vi "Mouse Move.vi"(7 "Map Model in":refnum<class "Map Model.lvclass">, 8 "error in (no error)":errorcluster, 10 "Position":T1, 11 "Pencil in":refnum<class "Pencil.lvclass">) -> (0 "error out":errorcluster, 3 "Pencil out":refnum<class "Pencil.lvclass">, 5 "Map Model out":refnum<class "Map Model.lvclass">)   [LabVIEW 2020, in "Map Model.lvlib" / "Pencil.lvclass"]
uses:
  Pencil.lvclass
  E:/Project/Labview-Projects/Completed projects/Map Editor/Models/Map Model/Tools/Tool/Tool.lvclass
  <vilib>/Utility/miscctls.llb/LVPoint32TypeDef.ctl
  Map Model/Map Model.lvclass
  Tool/Tool.lvclass/Tool.ctl
  Map Model/Map Model.lvclass/Map Model.ctl
  Undoable Tool/Undoable Tool.lvclass
  Tool/Tool.lvclass
panel:
  # "NOTICE -- YOU MUST LEAVE THIS NOTICE IN PLACE.\n\nCopyright (c) 2017, LIANG LIU Shawn.Liu.cn@gmail.com\nAll rights reserved.\n\nRedistribution and use in source and binary forms, with or without modification, are permitted provided that the following conditions are met:\n-Redistributions of source code must retain the above copyright notice, this list of conditions and the following disclaimer.\n-Redistributions in binary form must reproduce the above copyright notice, this list of conditions and the following disclaimer in the documentation and/or other materials provided with the distribution.\n-Neither the name of the eLp nor the names of its contributors may be used to endorse or promote products derived from this software without specific prior written permission.\n\nTHIS SOFTWARE IS PROVIDED BY THE COPYRIGHT HOLDERS AND CONTRIBUTORS \"AS IS\" AND ANY EXPRESS OR IMPLIED WARRANTIES, INCLUDING, BUT NOT LIMITED TO, THE IMPLIED WARRANTIES OF MERCHANTABILITY AND FITNESS FOR A PARTICULAR PURPOSE ARE DISCLAIMED. IN NO EVENT SHALL THE COPYRIGHT HOLDER OR CONTRIBUTORS BE LIABLE FOR ANY DIRECT, INDIRECT, INCIDENTAL, SPECIAL, EXEMPLARY, OR CONSEQUENTIAL DAMAGES (INCLUDING, BUT NOT LIMITED TO, PROCUREMENT OF SUBSTITUTE GOODS OR SERVICES; LOSS OF USE, DATA, OR PROFITS; OR BUSINESS INTERRUPTION) HOWEVER CAUSED AND ON ANY THEORY OF LIABILITY, WHETHER IN CONTRACT, STRICT LIABILITY, OR TORT (INCLUDING NEGLIGENCE OR OTHERWISE) ARISING IN ANY WAY OUT OF THE USE OF THIS SOFTWARE, EVEN IF ADVISED OF THE POSSIBILITY OF SUCH DAMAGE."
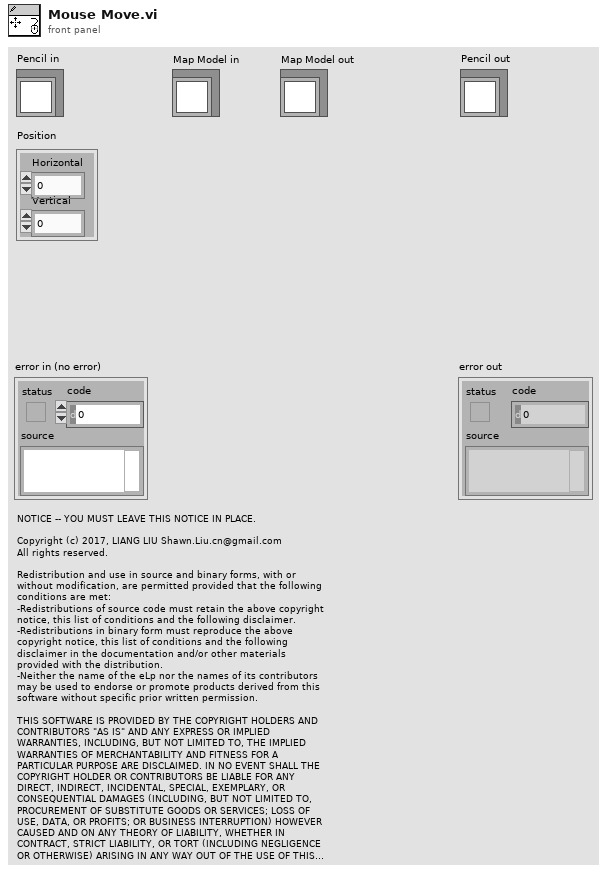
[diagram p1: front panel]
types:
  T1 = typedef "LVPoint32TypeDef.ctl" = cluster{"Horizontal":i32, "Vertical":i32}
  T2 = cluster{"Width":u16, "Style":enum32{"Solid", "Dash", "Dot", "DashDot", "DashDotDot"}}
  T3 = cluster{"Occupied Color":cluster{"Value":u8, "Color":u32}, "Free Color":cluster{"Value":u8, "Color":u32}, "Unknown Color":cluster{"Value":u8, "Color":u32}}
  T4 = typedef "LVPointTypeDef.ctl" = cluster{"Horizontal":i16, "Vertical":i16}
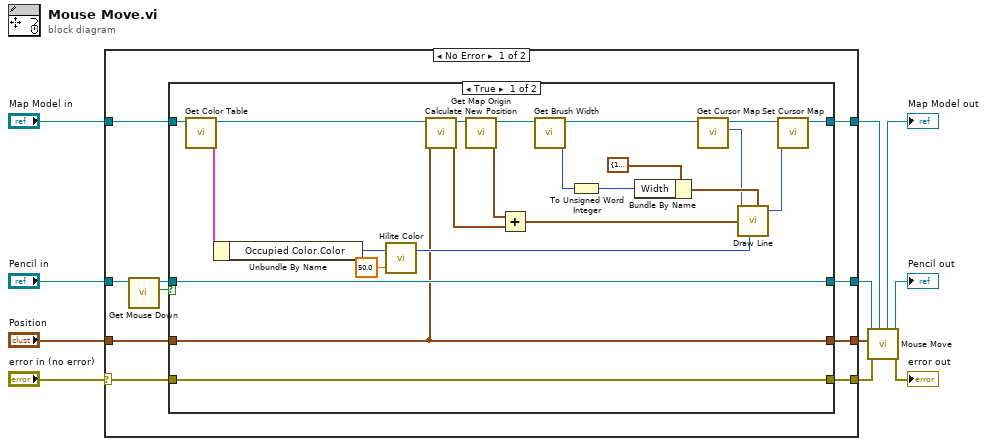
[diagram p0: block diagram]
diagram:
  n1 = case shown="No Error" "error in (no error)" {
    selector: "error in (no error)" -> [w18 w52]
    tunnel: "Map Model in" -> [w21 w51]
    tunnel: [w20 w51] -> w8
    tunnel: [w19 w49] -> w7
    tunnel: "Position" -> [w17 w49]
    tunnel: "Pencil in" -> [w16 w50]
    tunnel: [w15 w50] -> w3
    tunnel: [w14 w52] -> w2
    frame No Error {
      n2 = call "Get Mouse Down.vi"("Tool in"=w16) -> ("Mouse Down"=w12:bool, "Tool out"=w13:refnum<class "Pencil.lvclass">)  [unwired: 9 in]
      n3 = case shown="True" w12 {
        tunnel: w13 -> [w44 w48]
        tunnel: w21 -> [w43 w45]
        tunnel: [w22 w45] -> w20
        tunnel: [w44 w48] -> w15
        tunnel: w17 -> [w23 w46]
        tunnel: [w23 w46] -> w19
        tunnel: w18 -> [w33 w47]
        tunnel: [w33 w47] -> w14
        frame True {
          n4 = call "Get Color Table.vi"("Map Model in"=w43) -> ("Color Table"=w37:T3, "Map Model out"=w38:refnum<class "Map Model.lvclass">)  [unwired: 9 in]
          n5 = Unbundle By Name(w37) -> ("Occupied Color.Color"=w36:u32)
          n6 = call <vilib>:"Hilite Color.vi"("Percentage(30)"=50.0, "Color In"=w36) -> ("Hilite"=w30:u32)  [unwired: 1 out]
          n7 = call "Calculate New Position.vi"("Position in"=w23, "Map Model in"=w38) -> ("Position out"=w24:T1, "Map Model out"=w25:refnum<class "Map Model.lvclass">)  [unwired: 8 in]
          n8 = call "Get Map Origin.vi"("Map Model in"=w25) -> ("Map Origin"=w31:T4, "Map Model out"=w32:refnum<class "Map Model.lvclass">)  [unwired: 9 in]
          n9 = Add(x=w31, y=w24) -> (x+y=w28:T1)
          n10 = call "Get Brush Width.vi"("Map Model in"=w32) -> ("Brush Width"=w35:i32, "Map Model out"=w41:refnum<class "Map Model.lvclass">)  [unwired: 9 in]
          n11 = To Unsigned Word Integer(number=w35) -> (unsigned 16bit integer=w34:u16)
          n12 = Bundle By Name(cluster=T2 {"Width"=1, "Style"=enum."Solid"} ("pen"), "Width"=w34) -> (w39:T2)
          n13 = call "Get Cursor Map.vi"("Map Model in"=w41) -> ("Cursor Map"=w26:picture, "Map Model out"=w27:refnum<class "Map Model.lvclass">)  [unwired: 9 in]
          n14 = call <vilib>:"Draw Line.vi"("picture"=w26, "end point"=w28, "color(black)"=w30, "pen"=w39) -> ("new picture"=w42:picture)  [unwired: 5 in]
          n15 = call "Set Cursor Map.vi"("Cursor Map"=w42, "Map Model in"=w27) -> ("Map Model out"=w22:refnum<class "Map Model.lvclass">)  [unwired: 9 in]
        }
        frame False {
        }
      }
    }
    frame Error {
    }
  }
  n16 = call-parent "Mouse Move.vi"("Map Model in"=w8, "error in (no error)"=w2, "Position"=w7, "Tool in"=w3) -> ("error out"=→"error out":errorcluster, "Tool out"=→"Pencil out":refnum<class "Pencil.lvclass">, "Map Model out"=→"Map Model out":refnum<class "Map Model.lvclass">)  [unwired: 5 in]
